vi "Update-sequence.vi"(8 "error in (no error)":errorcluster, 11 "Object ref in":T1) -> (0 "error out":errorcluster, 3 "Object ref out":T1)   [LabVIEW 2013, in "PowderDeposition.lvlib" / "PD-Main.lvclass"]
uses:
  PD-Main.lvclass
  Object-reference.ctl
  PD-Main.lvclass/PD-Main.ctl
  Motor/Motor.lvclass
  Assembly/Motor-assembly.lvclass
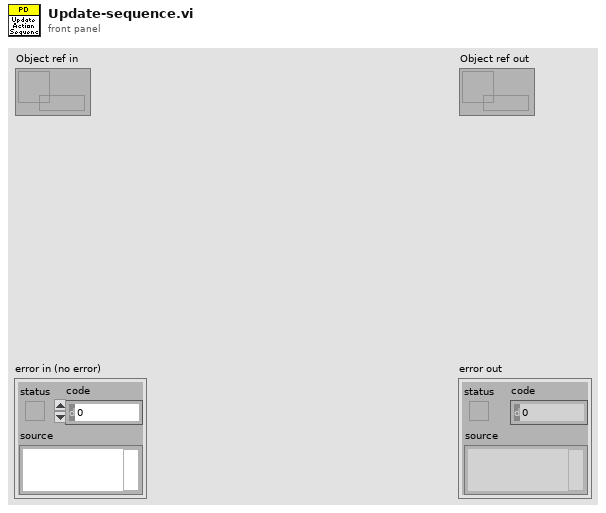
[diagram p1: front panel]
types:
  T1 = typedef "PowderDeposition.lvlib/PD-Main.lvclass/Object-reference.ctl" = refnum<data-value>
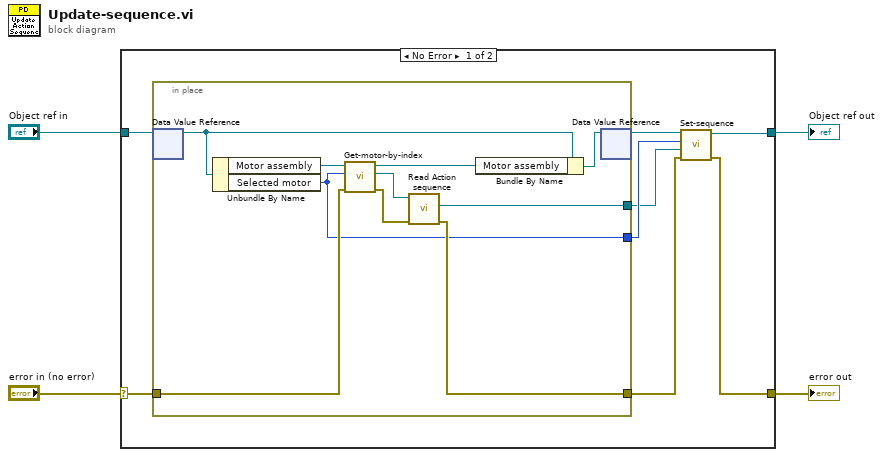
[diagram p0: block diagram]
diagram:
  n1 = case shown="No Error" "error in (no error)" {
    selector: "error in (no error)" -> [w11 w24]
    tunnel: [w7 w24] -> w3
    tunnel: [w8 w23] -> w1
    tunnel: "Object ref in" -> [w12 w23]
    frame No Error {
      n2 = in-place {
        in-place-border: [w14] -> w9
        in-place-border: w11 -> [w18]
        in-place-border: [w15] -> w5
        in-place-border: [w13] -> w6
        n3 = in-place-dvr #1(w12) -> (w22:refnum<class "PD-Main.lvclass">)  [unwired: 1 out]
        n4 = Unbundle By Name(w22) -> ("Motor assembly"=w20:refnum<class "Motor-assembly.lvclass">, "Selected motor"=w13:i32)
        n5 = call "Get-motor-by-index.vi"("error in (no error)"=w18, "Index"=w13, "Available motors in"=w20) -> ("error out"=w17:errorcluster, "Motor"=w16:refnum<class "Motor.lvclass">, "Available motors out"=w19:refnum<class "Motor-assembly.lvclass">)  [unwired: 5 in, 1 out]
        n6 = call-dynamic "Read Action sequence.vi"("error in (no error)"=w17, "Motor in"=w16) -> ("error out"=w14:errorcluster, "Sequence.lvclass"=w15:refnum<class "Action-sequence.lvclass">)  [unwired: 7 in, 1 out]
        n7 = Bundle By Name(cluster=w22, "Motor assembly"=w19) -> (w21:refnum<class "PD-Main.lvclass">)
        n8 = in-place-dvr #1(w21) -> (w10:T1)  [unwired: 1 out]
      }
      n9 = call "Set-sequence.vi"("error in (no error)"=w9, "Sequence"=w5, "Motor index"=w6, "Object ref in"=w10) -> ("error out"=w7:errorcluster, "Object ref out"=w8:T1)  [unwired: 6 in]
    }
    frame Error {
    }
  }
  "error out" <- w3
  "Object ref out" <- w1
